vi "Write.vi"(9 "array":u8[](array[numeric]), 10 "error in (no error)":errorcluster, 11 "FPGA VI Reference In":T1) -> (1 "Status":u8, 2 "error out":errorcluster, 3 "FPGA VI Reference Out":T1)   [LabVIEW 2016]
uses:
  FPGA Bitfiles/FPGA_defref.ctl
  <vilib>/Utility/error.llb/Error Cluster From Error Code.vi
  <vilib>/rvi/errors/niLvFpgaAdjustHostInterfaceError.vi
  <vilib>/rvi/interface/nirviReadWriteControl/nirviReadWriteControl.xnode
  FPGA Bitfiles/nRF24Communicati_FPGATarget_FPGATest_lnf7SjQfCOM.lvbitx
  FPGATest.vi
  NiFpgaLv.dll
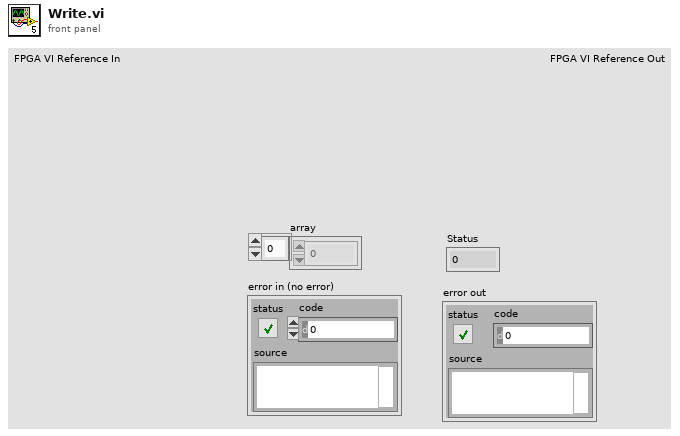
[diagram p1: front panel]
types:
  T1 = typedef "FPGA_defref.ctl" = refnum<k20>
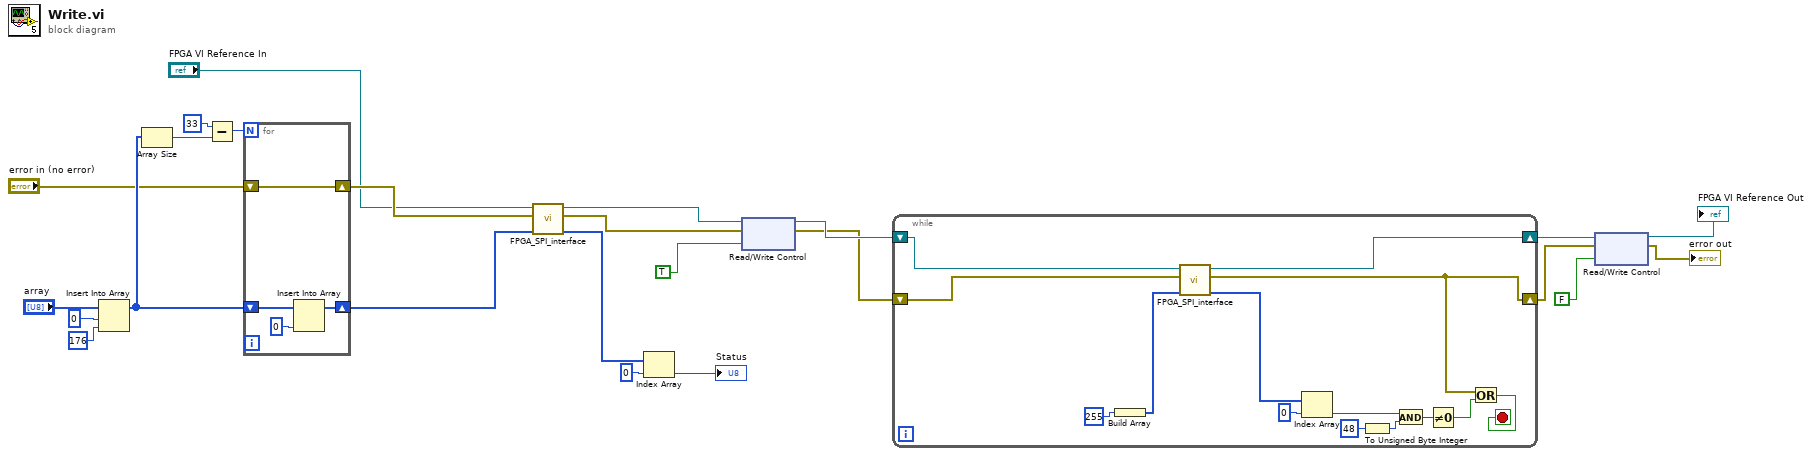
[diagram p0: block diagram]
diagram:
  n1 = Insert Into Array(array="array", index=0, new element=176) -> (w16:u8[])
  n2 = Array Size(array=w16) -> (size(s)=w19:i32)
  n3 = Subtract(x=33, y=w19) -> (x-y=w18:i32)
  n4 = for {
    N: w18 -> [_]
    shift-right: [w27] -> w13
    shift-left: w16 -> [w28]
    shift-right: [w25] -> w14
    shift-left: "error in (no error)" -> [w25]
    n5 = Insert Into Array(array=w28, new element=0 ("new element/subarray")) -> (w27:u8[])  [unwired: 1 in]
  }
  n6 = call "FPGA_SPI_interface.vi"("Frames to Write"=w13, "error in"=w14, "FPGA VI Reference In"="FPGA VI Reference In") -> ("Frames Read"=w12:u8[], "error out"=w10:errorcluster, "FPGA VI Reference Out"=w11:T1)  [unwired: 6 in]
  n7 = Index Array(array=w12, index=0) -> (element=→"Status":u8)
  n8 = xnode "Read/Write Control"("FPGA VI Reference In"=w11, "error in"=w10, "CE"=TRUE ("SPI/CS1 (Pin 4)")) -> ("FPGA VI Reference Out"=w9:T1, "error out"=w8:errorcluster)
  n9 = while {
    shift-right: [w30] -> w5
    shift-left: w8 -> [w38]
    shift-right: [w34] -> w6
    shift-left: w9 -> [w35]
    stop <- w31 stop-if-true
    n10 = Build Array(255) -> (w37:i32[])
    n11 = call "FPGA_SPI_interface.vi"("Frames to Write"=w37, "error in"=w38, "FPGA VI Reference In"=w35) -> ("Frames Read"=w36:u8[], "error out"=w30:errorcluster, "FPGA VI Reference Out"=w34:T1)  [unwired: 6 in]
    n12 = Index Array(array=w36, index=0) -> (element=w41:u8)
    n13 = To Unsigned Byte Integer(number=48 ("x")) -> (unsigned 8bit integer=w32:u8)
    n14 = And(x=w41, y=w32) -> (x .and. y?=w39:u8)
    n15 = Not Equal To 0?(x=w39) -> (x != 0?=w29:bool)
    n16 = Or(x=w30, y=w29) -> (x .or. y?=w31:bool)
  }
  n17 = xnode "Read/Write Control"("FPGA VI Reference In"=w6, "error in"=w5, "CE"=FALSE ("SPI/CS1 (Pin 4)")) -> ("FPGA VI Reference Out"=→"FPGA VI Reference Out":T1, "error out"=→"error out":errorcluster)
